vi "Set Aperture Time.vi"(0 "reference":refnum<k15>, 5 "Aperture Time(s)":dbl=0.3 format="%#_6p", 9 "Number of Averages":dbl=1.0, 11 "error in (no error)":errorcluster) -> (4 "reference out":refnum<k15>, 15 "error out":errorcluster)   [LabVIEW 2023, in "NI-568x RF Power Meter.lvlib" / "SG 2250 Path Accessor.lvclass"]
uses:
  SG 2250 Path Accessor.lvclass
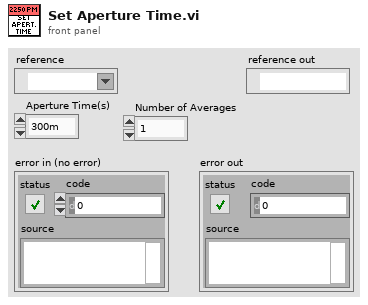
[diagram p1: front panel]
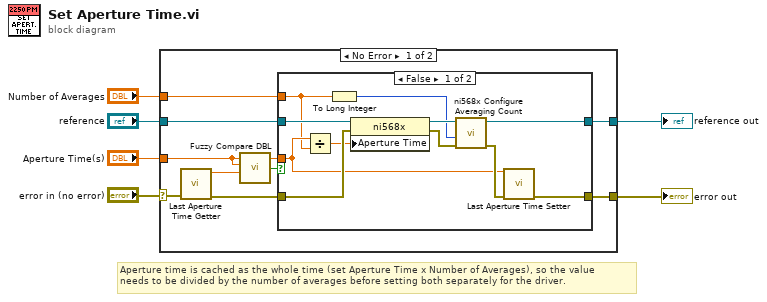
[diagram p0: block diagram]
diagram:
  # "Aperture time is cached as the whole time (set Aperture Time x Number of Averages), so the value\nneeds to be divided by the number of averages before setting both separately for the driver."
  n1 = case shown="No Error" "error in (no error)" {
    selector: "error in (no error)" -> [w15 w29]
    tunnel: "reference" -> [w11 w30]
    tunnel: [w10 w29] -> w5
    tunnel: [w9 w30] -> w4
    tunnel: "Aperture Time(s)" -> [w8 _]
    tunnel: "Number of Averages" -> [w7 _]
    frame No Error {
      n2 = call "Last Aperture Time Getter.vi"("error in (no error)"=w15) -> ("Aperture Time (s)"=w14:dbl, "error out"=w13:errorcluster)  [unwired: 13 in]
      n3 = call "Fuzzy Compare DBL.vi"("A"=w8, "B"=w14) -> ("Fuzzy Equal?"=w12:bool)  [unwired: 5 in]
      n4 = case shown="False" w12 {
        tunnel: w13 -> [w25 w28]
        tunnel: w11 -> [w24 w27]
        tunnel: [w26 w28] -> w10
        tunnel: [w22 w27] -> w9
        tunnel: w8 -> [w18 _]
        tunnel: w7 -> [w17 _]
        frame False {
          n5 = Divide(x=w18, y=w17) -> (x/y=w16:dbl)
          n6 = To Long Integer(number=w17) -> (32bit integer=w19:i32)
          n7 = property class="ni568x"(reference=w24, error in=w25, "Aperture Time"=w16) -> (reference out=w23:refnum<k15>, error out=w21:errorcluster)
          n8 = call <instrlib>:"ni568x Configure Averaging Count.vi"("error in"=w21, "averaging count"=w19, "instrument handle"=w23) -> ("error out"=w20:errorcluster, "instrument handle out"=w22:refnum<k15>)  [unwired: 7 in]
          n9 = call "Last Aperture Time Setter.vi"("Aperture Time (s)"=w18, "error in (no error)"=w20) -> ("error out"=w26:errorcluster)  [unwired: 13 in]
        }
        frame True {
        }
      }
    }
    frame Error {
    }
  }
  "error out" <- w5
  "reference out" <- w4
